vi "CSH.vi"(10 "数组":i32[](array[numeric]), 11 "hDevice输入":i32) -> (2 "数值":i32, 3 "hDevice输出":i32)   [LabVIEW 2012]
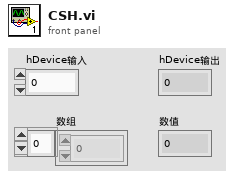
[diagram p1: front panel]
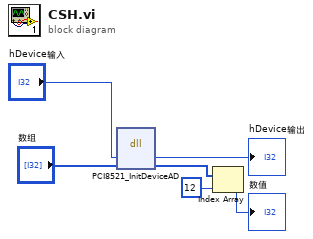
[diagram p0: block diagram]
diagram:
  n1 = dll-call lib="PCI8521_32" fn="PCI8521_InitDeviceAD" label="InitDeviceAD"("hDevice"="hDevice输入", "pADPara"="数组") -> ("hDevice"=→"hDevice输出":i32, "pADPara"=w5:i32[])  [unwired: 4 in, 2 out]
  n2 = Index Array(array=w5, index=12) -> (element=→"数值":i32)
